vi "GetOneOfAccessorList.vi"() -> (0 "Array":string[](array[string]))   [LabVIEW 2019, in "gRPC Template Creation Utility.lvlib"]
uses:
  gRPC Template Creation Utility.lvlib
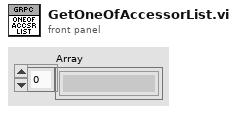
[diagram p1: front panel]
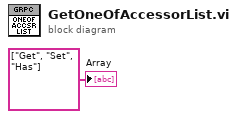
[diagram p0: block diagram]
diagram:
  "Array" <- string[] ["Get", "Set", "Has"]
